vi "TDMS Logger.vi"() -> ()   [LabVIEW 2012]
uses:
  <vilib>/Utility/error.llb/Error Cluster From Error Code.vi
  <vilib>/ErrorRing/Error Ring.xnode
panel:
  out "功率谱":waveform(dbl)[](graph)
  out "时间数据":waveform(dbl)[](graph)
  in  "UUT序列号":string[](array[string])
  in  "测试操作员":string
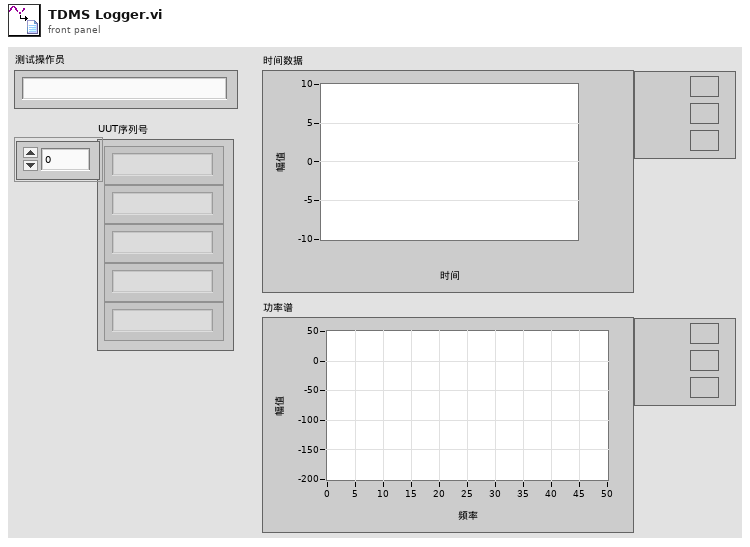
[diagram p1: front panel]
types:
  T1 = enum16{"open", "open or create", "create or replace", "create", "open (read-only)"}
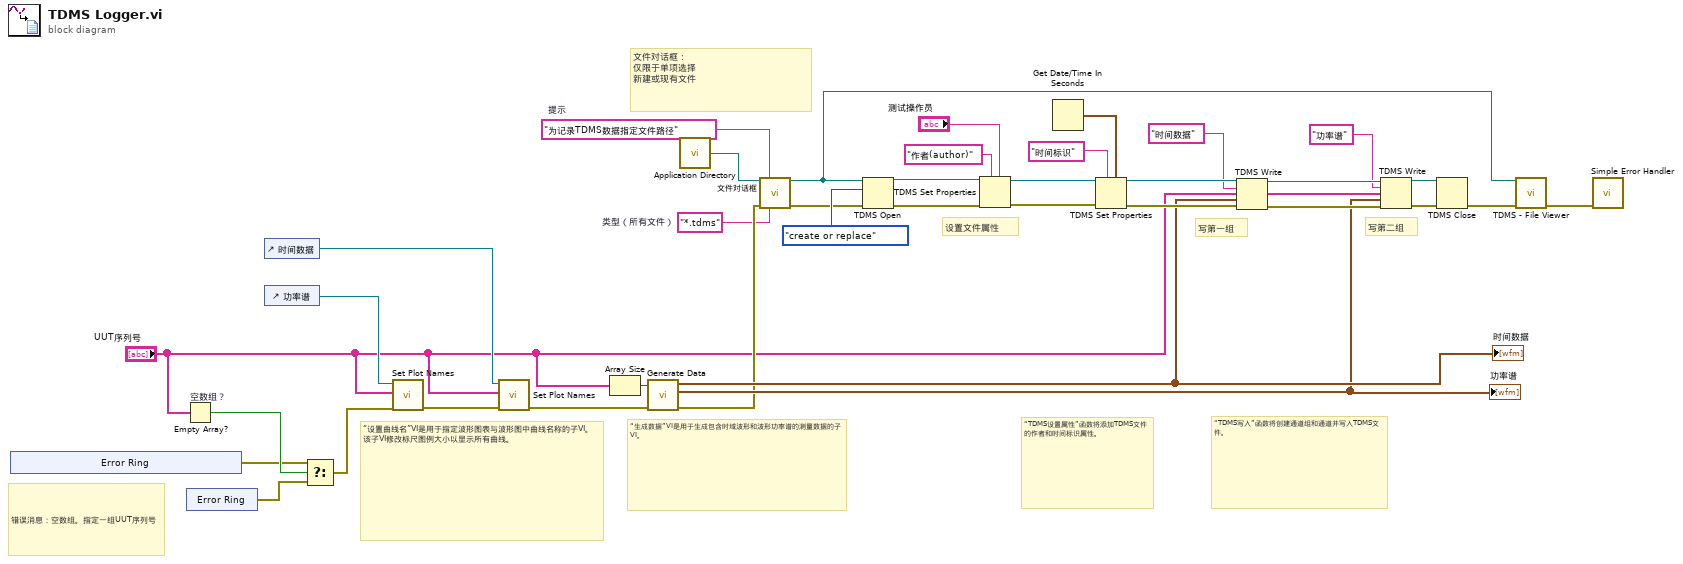
[diagram p0: block diagram]
diagram:
  w8 = "*.tdms"  # 类型（所有文件）
  w12 = "为记录TDMS数据指定文件路径"  # 提示
  # "错误消息：空数组。指定一组UUT序列号"
  # "文件对话框：\n仅限于单项选择\n新建或现有文件"
  # "写第二组"
  # "写第一组"
  # "设置文件属性"
  # "“TDMS设置属性”函数将添加TDMS文件的作者和时间标识属性。"
  # "“TDMS写入”函数将创建通道组和通道并写入TDMS文件。"
  # "“生成数据”VI是用于生成包含时域波形和波形功率谱的测量数据的子VI。"
  # "“设置曲线名”VI是用于指定波形图表与波形图中曲线名称的子VI。\n该子VI修改标尺图例大小以显示所有曲线。"
  n1 = xnode "Error Ring"() -> ("错误输出"=w1:errorcluster)
  n2 = Empty Array? "空数组？"(array="UUT序列号") -> (empty?=w5:bool)
  n3 = xnode "Error Ring"() -> ("错误输出"=w2:errorcluster)
  n4 = control-ref of="时间数据"() -> (w14:refnum<vi>)
  n5 = control-ref of="功率谱"() -> (w15:refnum<vi>)
  n6 = Select ("选择")(t=w1, s=w5, f=w2) -> (s? t:f=w3:errorcluster)
  n7 = call "Set Plot Names.vi"("错误输入"=w3, "曲线名"="UUT序列号", "图形引用"=w15) -> ("错误输出"=w38:cluster{"状态":bool, "代码":i32, "源":string})  [unwired: 8 in]
  n8 = call "Set Plot Names.vi"("错误输入"=w38, "曲线名"="UUT序列号", "图形引用"=w14) -> ("错误输出"=w4:cluster{"状态":bool, "代码":i32, "源":string})  [unwired: 8 in]
  n9 = Array Size ("数组大小")(array="UUT序列号") -> (size(s)=w37:i32)
  n10 = call "Generate Data.vi"("错误输入"=w4, "通道数"=w37) -> ("错误输出"=w10:cluster{"状态":bool, "代码":i32, "源":string}, "功率谱"=w16:waveform(dbl)[], "时间数据"=w17:waveform(dbl)[])  [unwired: 7 in]
  "时间数据" <- w17
  "功率谱" <- w16
  n11 = call <vilib>:"Application Directory.vi"() -> ("Application Directory"=w11:path)
  n12 = call "文件对话框"("start path"=w11, "prompt"=w12, "error in"=w10, "pattern (all files)"=w8) -> ("selected path"=w13:path, "error out"=w9:errorcluster)  [unwired: 8 in, 2 out]
  n13 = TDMS Open ("TDMS打开")(8:w9, 10:T1."create or replace" ("操作(0:open)"), 11:w13) -> (0:w30:errorcluster, 3:w35:refnum<k34>)  [unwired: 3 in]
  n14 = TDMS Set Properties ("TDMS设置属性")(5:"测试操作员", 7:"作者(author)", 8:w30, 11:w35) -> (0:w34:errorcluster, 3:w33:refnum<k34>)  [unwired: 2 in, 2 out]
  n15 = Get Date/Time In Seconds ("获取日期/时间（秒）")() -> (seconds since 1Jan1904=w31:timestamp)
  n16 = TDMS Set Properties ("TDMS设置属性")(5:w31, 7:"时间标识" ("标题"), 8:w34, 11:w33) -> (0:w28:errorcluster, 3:w29:refnum<k34>)  [unwired: 2 in, 2 out]
  n17 = TDMS Write ("TDMS写入")(0:w29, 5:"时间数据" ("组名称输入（无标题）"), 7:"UUT序列号", 9:w17, 11:w28) -> (4:w26:refnum<k34>, 8:w23:string[], 15:w25:errorcluster)  [unwired: 1 in, 1 out]
  n18 = TDMS Write ("TDMS写入")(0:w26, 5:"功率谱" ("组名称输入（无标题）"), 7:w23, 9:w16, 11:w25) -> (4:w22:refnum<k34>, 15:w21:errorcluster)  [unwired: 1 in, 2 out]
  n19 = TDMS Close ("TDMS关闭")(8:w21, 11:w22) -> (0:w20:errorcluster)  [unwired: 1 out]
  n20 = call <vilib>:"TDMS - File Viewer.vi"("error in (no error)"=w20, "file path"=w13) -> ("error out"=w19:errorcluster)  [unwired: 4 in, 1 out]
  n21 = call <vilib>:"Simple Error Handler.vi"("error in (no error)"=w19) -> ()  [unwired: 4 in, 5 out]
